vi "valve.vi"(8 "error in":errorcluster, 10 "ON":bool=TRUE, 11 "Valve":u16=999) -> (0 "error out":errorcluster)   [LabVIEW 2013]
uses:
  GlobalVariables/ValveParameters.vi
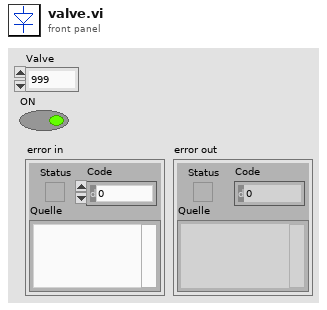
[diagram p1: front panel]
types:
  T1 = cluster{"baudrate":u32, "databits":u16, "paritybit":u16, "stopbits":u16, "flux control":u16, "Port":string, "Serial Parameters":cluster{"Mode":enum16{"RTU", "ASCII"}, "Slave Address":u8}, "Timeout":u32, "Valve mapping":cluster{"Inlet Valve":u8, "V1":u8, "V2":u8, "Sample Valve":u8, "Outlet Valve":u8}}
  T2 = cluster{"Mode":enum16{"RTU", "ASCII"}, "Slave Address":u8}
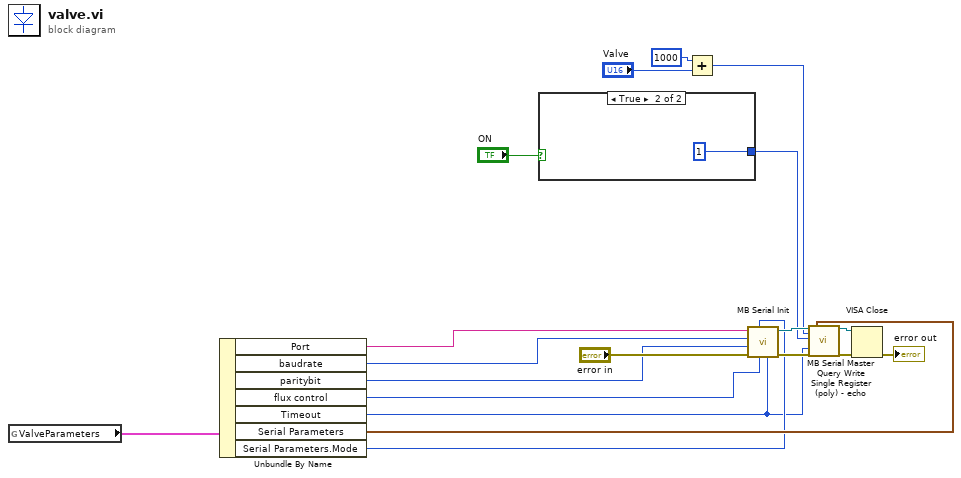
[diagram p0: block diagram]
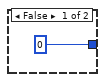
[diagram p2: hidden frame]
diagram:
  n1 = global read "ValveParameters.vi" "ValveParameters"() -> (w9:T1)
  n2 = Unbundle By Name(w9) -> ("Port"=w7:string, "baudrate"=w6:u32, "paritybit"=w5:u16, "flux control"=w4:u16, "Timeout"=w1:u32, "Serial Parameters"=w3:T2, "Serial Parameters.Mode"=w2:enum16{"RTU", "ASCII"})
  n3 = case shown="True" "ON" {
    tunnel: [u16 0 ("Register") u16 1 ("Register")] -> w11
    frame False {
    }
    frame True {
    }
  }
  n4 = Add(x=u16 1000 ("Address"), y="Valve") -> (x+y=w10:u16)
  n5 = call "MB Serial Init.vi"("Timeout"=w1, "Flow Control"=w4, "Mode"=w2, "error in (no error)"="error in", "Parity"=w5, "Baud Rate"=w6, "VISA resource name"=w7) -> ("error out"=w13:errorcluster, "VISA resource name out"=w12:refnum<visa-resource-name>)  [unwired: 3 out]
  n6 = call "MB Serial Master Query Write Single Register (poly) - echo.vi"("VISA resource name"=w12, "Address"=w10, "Holding Register"=w11, "Timeout"=w1, "error in"=w13, "Serial Parameters"=w3) -> ("VISA resource name out"=w14:refnum<visa-resource-name>, "error out"=w15:errorcluster)  [unwired: 11 in, 1 out]
  n7 = VISA Close(VISA resource name=w14, error in (no error)=w15) -> (error out=→"error out":errorcluster)
